vi "IV_Sweep_program1.vi"() -> ()   [LabVIEW 2013]
doc: "I. Description:\nThis example demonstrates how to continuously acquire and generate data at the same time, synchronized with one another.\n\nII. Instructions for Running:\n1. Select the physical channel to correspond to where your signal is input on the DAQ device. Also, select the corresponding channel for where your signal is being generated.\n2. Enter the minimum and maximum voltage ranges.\nNote: For better accuracy try to match the input range to the expected voltage level of the measured signal.\n3. Set the sample rate of the acquisition.\nNote: The rate should be at least twice as fast as the maximum frequency component of the signal being acquired. \n6. Select the Rate for the generation\n7. Select what type of signal to generate and the amplitude.\nNote: This example requires two DMA channels to run. If your hardware does not support two DMA channels, you need to set the Data Transfer Mechanism property for the Analog Output Task to use \"Interrupts\". The Data Transfer Mechanism property is located in the DAQmx Channel Property hierarchy at:\n\nDAQmx Channel Property Node>>Analog Output>>General Properties>>Advanced>>Data Transfer and Memory>>Data Transfer Mechanism\n\nRefer to your device documentation to determine how many DMA channels are supported for your hardware.\n\nIII. Block Diagram Steps:\n1. Create an analog input voltage channel. Also, create an analog output voltage channel.\n2. Set the rate for the sample clock. Additionally, define the sample mode to be continuous. Also, set the sample clock rate for the signal generation.\n2a. Call the Get Terminal Name with Device Prefix VI. This will take a Task and a terminal and create a properly formatted device + terminal name to use as the source of the Trigger.\n3. Define the parameters for a Digital Edge Start Trigger. Set the Analog output to trigger off the AI Start Trigger. This is an internal trigger signal.\n4. Use the Basic Function Generator VI to create the signal to be generated.\n5. Call the Start VI to arm the two functions. Make sure the analog output is armed before the analog input. This will ensure both will start at the same time.\n6. Read the waveform data in a loop until the user hits the stop button or an error occurs. The Is Task Done? VI is used to check for errors in the Analog Output Task.\n7. Call the Clear VI to Clear the Task\n8. Use the popup dialog box to display an error if any.\n\nIV. I/O Connections Overview:\nMake sure your signal input/output terminals match the Physical Channel I/O controls."
uses:
  <vilib>/Utility/error.llb/DialogType.ctl
  <vilib>/DAQmx/read.llb/DAQmx Read (Analog 1D DBL NChan 1Samp).vi
  <vilib>/DAQmx/write.llb/DAQmx Write (Analog DBL 1Chan 1Samp).vi
  <vilib>/DAQmx/create/channels.llb/DAQmx Create Channel (AO-Voltage-Basic).vi
  <vilib>/DAQmx/create/channels.llb/DAQmx Create Channel (AI-Voltage-Basic).vi
  <vilib>/DAQmx/configure/timing.llb/DAQmx Timing (Sample Clock).vi
  <vilib>/DAQmx/miscellaneous.llb/DAQmx Fill In Error Info.vi
  <vilib>/Utility/file.llb/Write To Spreadsheet File (DBL).vi
  <vilib>/Utility/file.llb/Write To Spreadsheet File (I64).vi
panel:
  out "Numeric":i32
  out "x/y":dbl
  in  "Sweep Amplitude":dbl=1.0
  in  "Stop Sweep":bool
  out "Connections 2":string="AI0=Current\nAI1=Bias\nAI2=dI/dV\nAI3=d2I/dV2\nAI4=X-Axis\nAI5=Z-Axis\n"
  out "Connections":string="AO0=Bias\nAO1=Z-axis\nAO2=X-Axis\nAO3=NA"
  in  "Columns":string
  out "Save Indicator":bool
  in  "Update Bias":bool
  in  "Save IV":bool
  in  "Save Decay":bool
  in  "Sweep Bias":bool
  in  "Step Z":bool
  in  "Comment":string="Molecule=C8\nGain=10nA\nBias Gain=div/1\nSweep Freq.=0.005Hz\nRef. Bias=5mV\nRef. Freq=4.33kHz\nGain LIA1=0.5mV\nTC LIA1=300ms\nGain LIA2=\nTC LIA2=\nLIA1=EGG"
  in  "Number Recorded":i32
  in  "DATA Filename":string="Data_"
  in  "Data Directory":path=path "E:/Research/Data"
  out "d2I/dV2":cluster{dbl[], dbl[]}(graph)
  out "dI/dV":cluster{dbl[], dbl[]}(graph)
  out "IV":cluster{dbl[], dbl[]}(graph)
  in  "# Samples":i32=2000
  in  "Frequency (Hz)":dbl=1.0
  in  "stop 3":bool
  in  "Bias":dbl caption="Bias Start Point" step=0.1 format="%_3g"
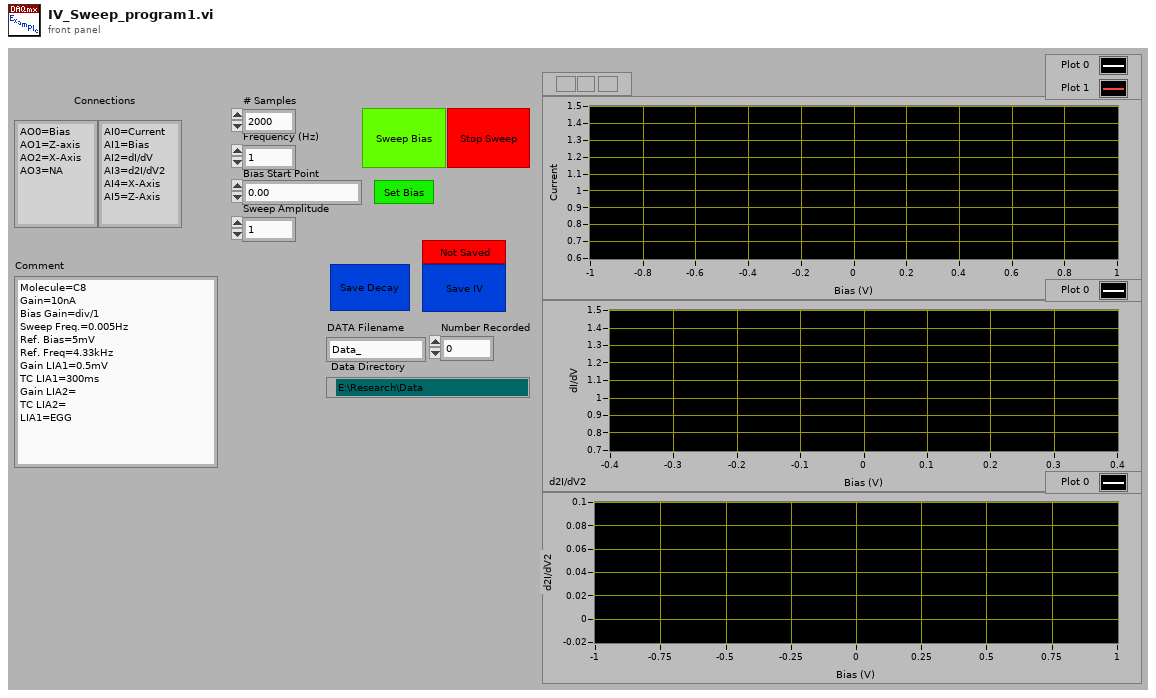
[diagram p1: front panel]
types:
  T1 = enum16{"open", "replace", "create", "open or create", "replace or create", "replace or create with confirmation"}
  T2 = typedef "DialogType.ctl" = u16
  T3 = cluster{dbl[], dbl[], dbl[], dbl[], dbl[], dbl[], dbl[]}
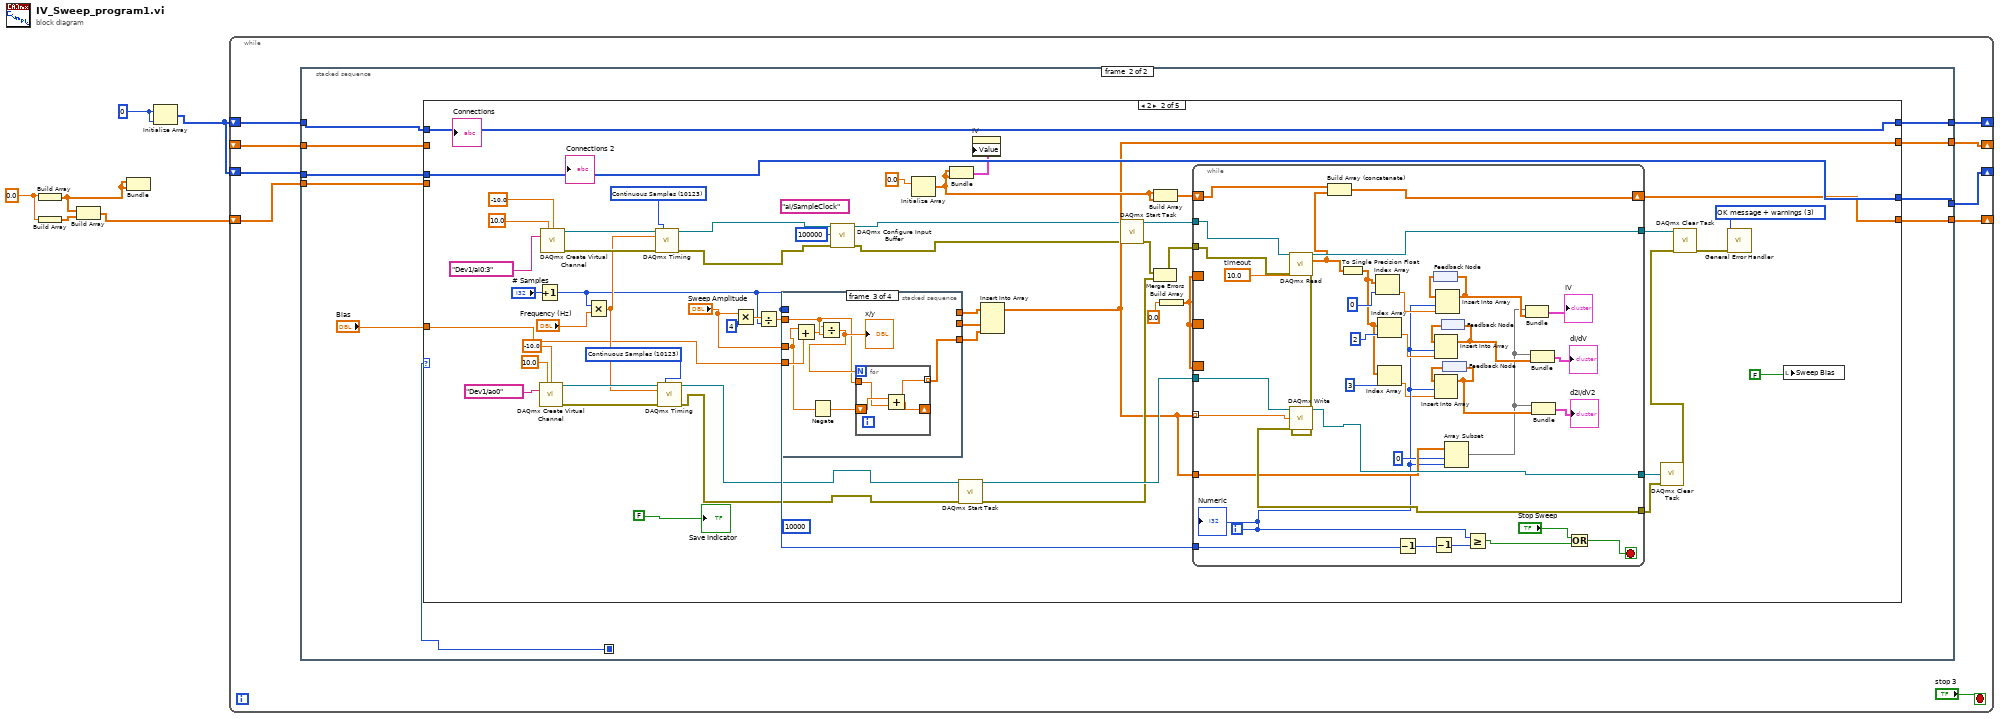
[diagram p0: block diagram]
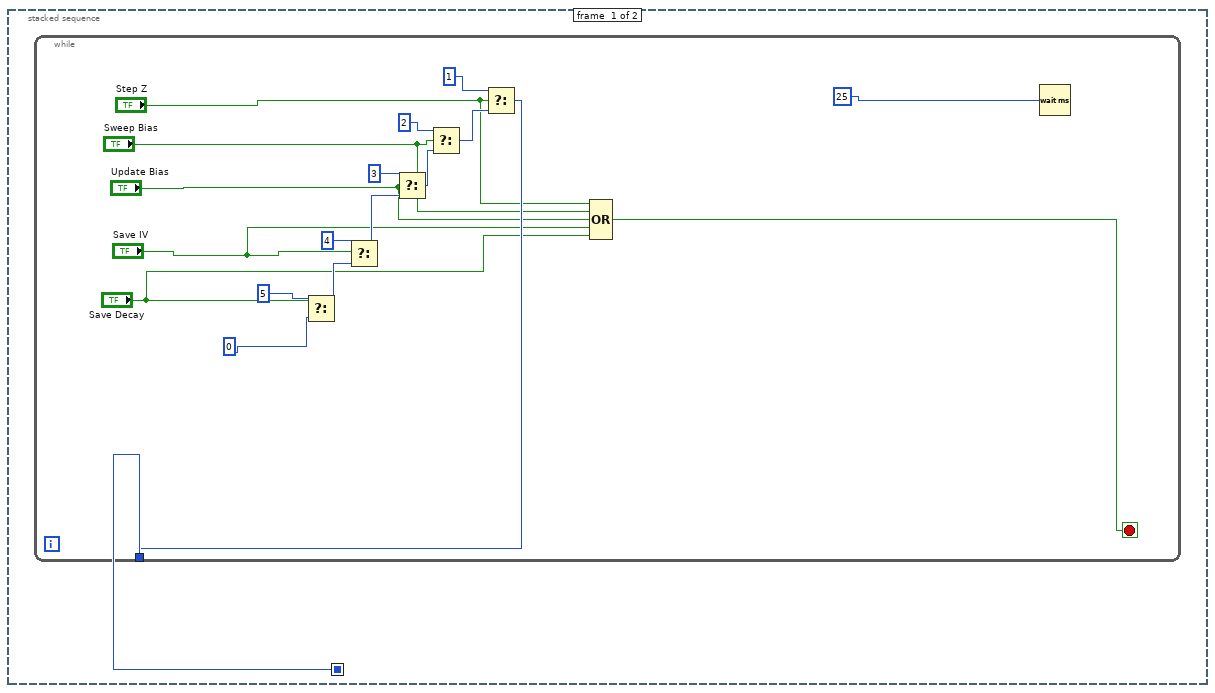
[diagram p2: hidden frame]
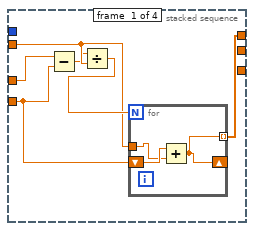
[diagram p4: hidden frame]
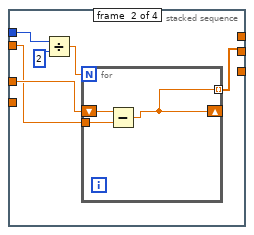
[diagram p5: hidden frame]
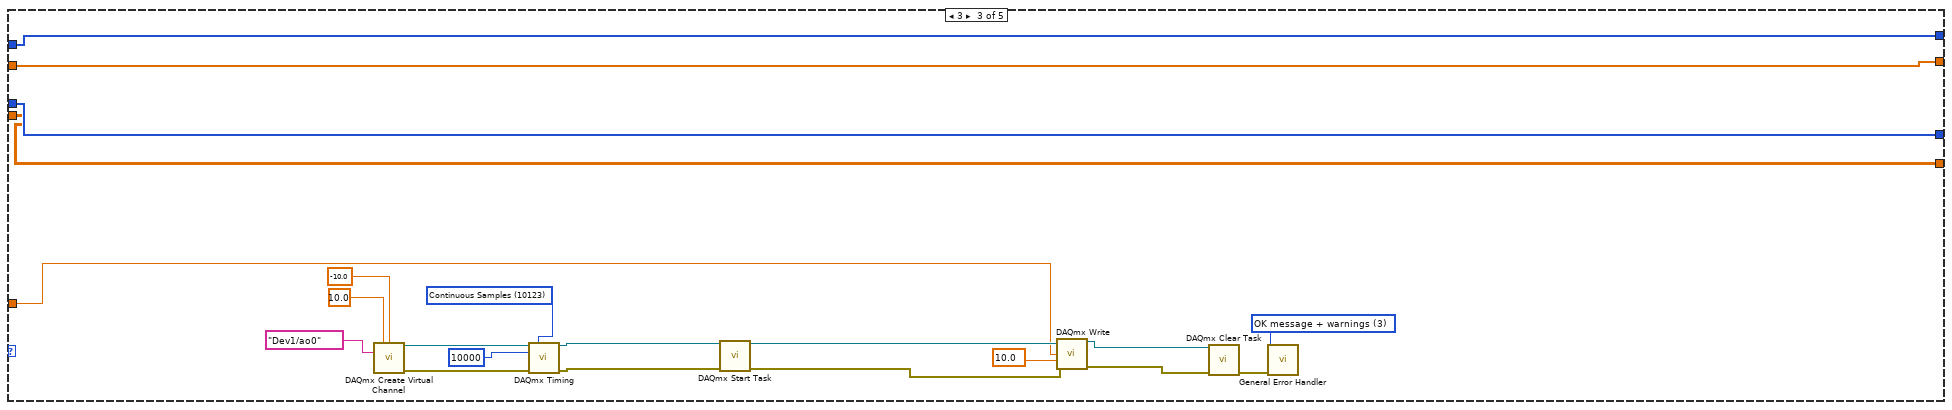
[diagram p7: hidden frame]
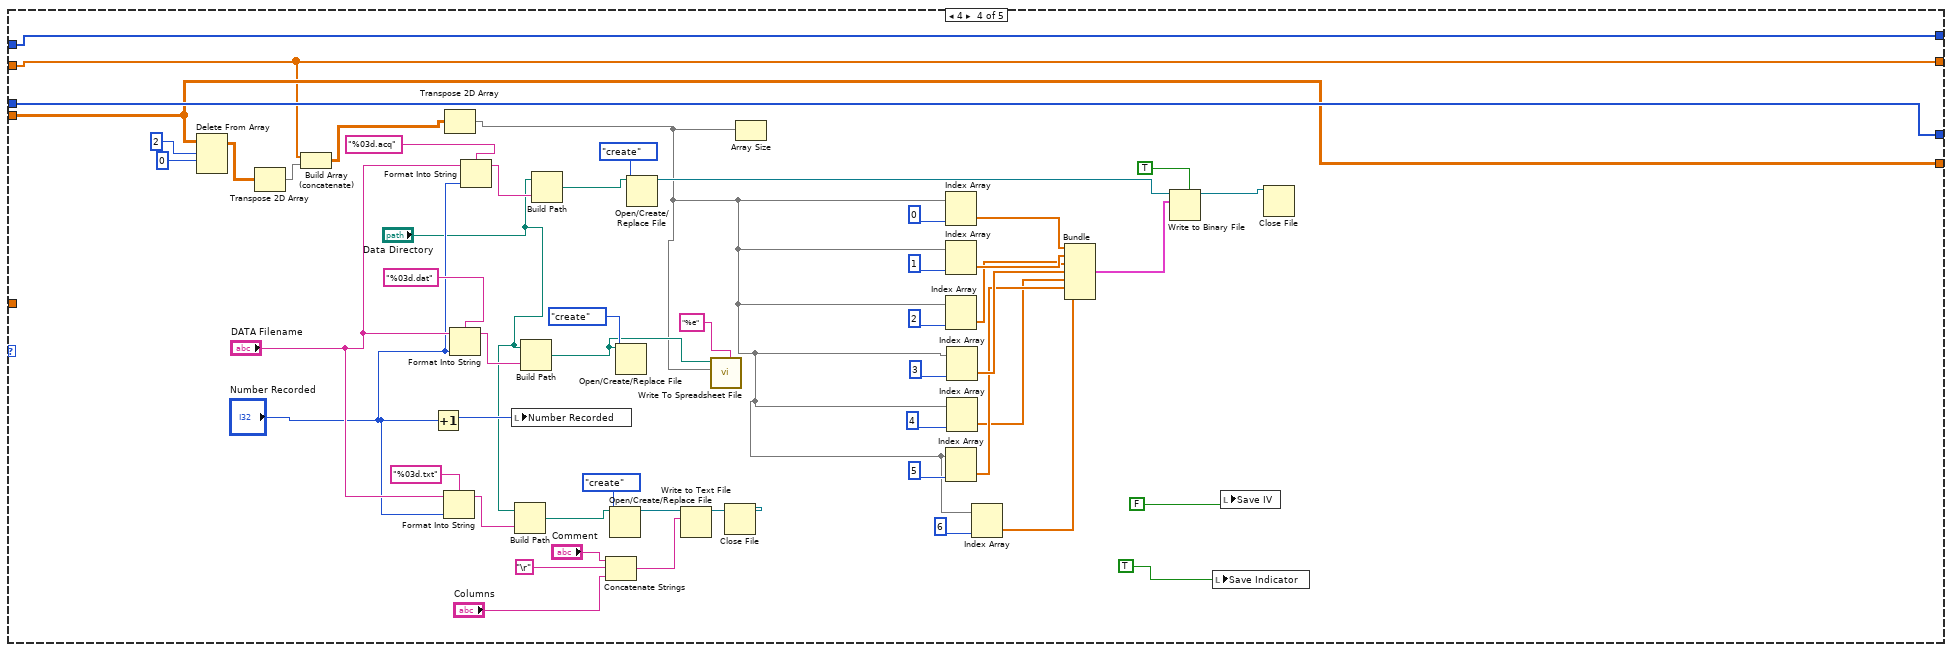
[diagram p8: hidden frame]
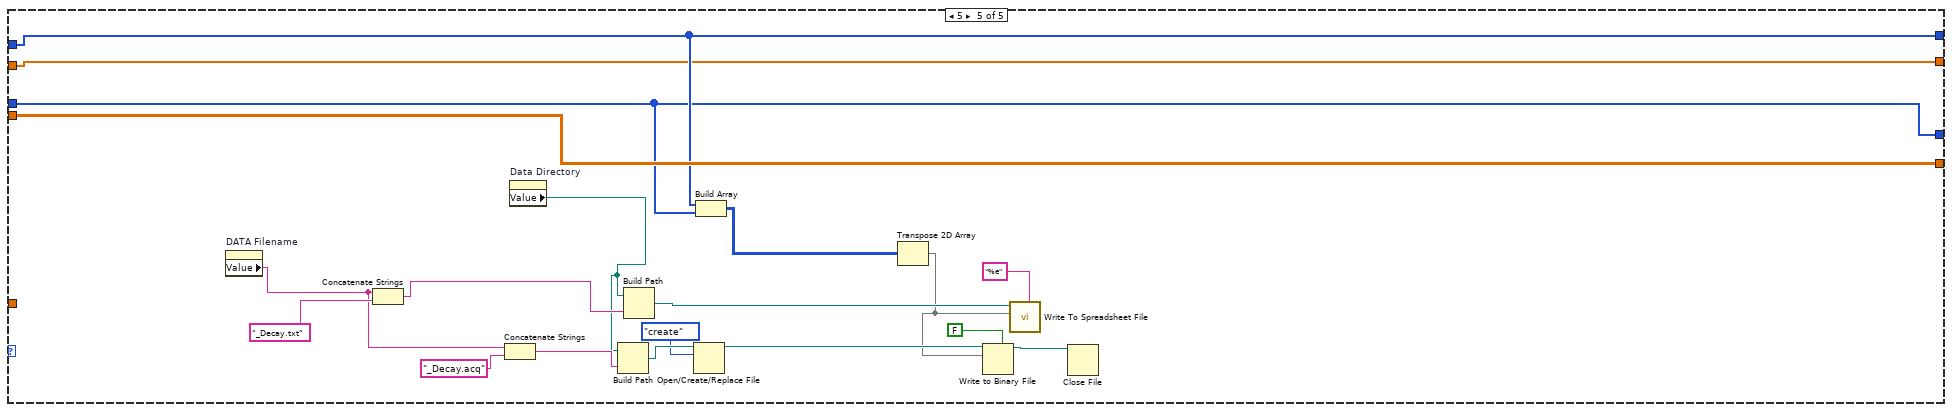
[diagram p9: hidden frame]
diagram:
  w2 = 0
  w6 = 0.0
  n1 = Build Array(w6) -> (w3:dbl[])
  n2 = Build Array(w6) -> (w5:dbl[])
  n3 = Build Array(w3, w5) -> (w4:dbl[][])
  n4 = Bundle(w3, w3) -> ()  [unwired: 1 in, 1 out]
  n5 = Initialize Array(w2, w2) -> (w1:i32[])
  n6 = while {
    shift-right: [w13] -> _
    shift-left: w1 -> [w14]
    shift-right: [w11] -> _
    shift-left: w1 -> [w12]
    shift-right: [w9] -> _
    shift-left: w4 -> [w10]
    shift-right: [w7] -> _
    shift-left: _ -> [w8]
    stop <- "stop 3" stop-if-true
    n7 = stacked-sequence {
      seq-local: [w16 _] -> [_ w44]
      tunnel: w14 -> [_ w43]
      tunnel: [_ w42] -> w13
      tunnel: w12 -> [_ w40]
      tunnel: [_ w39] -> w11
      tunnel: w10 -> [_ w38]
      tunnel: [_ w37] -> w9
      tunnel: w8 -> [_ w36]
      tunnel: [_ w35] -> w7
      frame #0 {
        n8 = while {
          tunnel: [w25] -> w16
          stop <- w24 stop-if-true
          n9 = Select(t=5, s="Save Decay", f=0) -> (s? t:f=w30:i32)
          n10 = Select(t=4, s="Save IV", f=w30) -> (s? t:f=w29:i32)
          n11 = Select(t=3, s="Update Bias", f=w29) -> (s? t:f=w27:i32)
          n12 = Select(t=2, s="Sweep Bias", f=w27) -> (s? t:f=w34:i32)
          n13 = Select(t=1, s="Step Z", f=w34) -> (s? t:f=w25:i32)
          n14 = Compound Arithmetic op=OR("Step Z", "Sweep Bias", "Update Bias", "Save IV", "Save Decay") -> (w24:bool)
          n15 = Wait (ms)(milliseconds to wait=25) -> ()  [unwired: 1 out]
        }
      }
      frame #1 {
        n16 = case shown="2" w44 {
          tunnel: w43 -> [w48 w86 w172 w237 w258]
          tunnel: [w48 w86 w172 w237 w258] -> w42
          tunnel: "Bias" -> [_ w72 w178 _ _]
          tunnel: w40 -> [w47 w83 w173 w238 w259]
          tunnel: [w47 w83 w173 w238 w259] -> w39
          tunnel: w38 -> [w46 _ w170 w217 w260]
          tunnel: [w46 w64 w170 w217 w260] -> w37
          tunnel: [w45 w56 w169 w215 w243] -> w35
          tunnel: w36 -> [w45 _ w169 w215 w243]
          frame 0, Default {
          }
          frame 2 {
            (unwired) 10000
            w81 = 10123 items=["Finite Samples"=10178, "Continuous Samples"=10123, "Hardware Timed Single Point"=12522] ("sample mode")
            w82 = 10123 items=["Finite Samples"=10178, "Continuous Samples"=10123, "Hardware Timed Single Point"=12522] ("sample mode")
            (unwired) "ai/SampleClock" ("terminal")
            w91 = T2 3 items=["no dialog", "OK message", "continue or stop message", "OK message + warnings", "continue/stop + warnings"] ("type of dialog (OK msg:1)")
            n17 = Increment(x="# Samples") -> (x+1=w62:i32)
            n18 = call-poly <vilib>:"DAQmx Create Virtual Channel.vi"("maximum value"=10.0, "minimum value"=-10.0, "physical channels"=tag "Dev1/ao0") -> ("task out"=w94:refnum<k21>, "error out"=w93:errorcluster)  [unwired: 11 in]
            n19 = call-poly <vilib>:"DAQmx Create Virtual Channel.vi"("maximum value"=10.0 ("Maximum Value"), "minimum value"=-10.0 ("Minimum Value"), "physical channels"=tag "Dev1/ai0:3" ("Physical Channel")) -> ("task out"=w98:refnum<k21>, "error out"=w99:errorcluster)  [unwired: 11 in]
            n20 = Multiply(x=w62, y="Frequency (Hz)") -> (x*y=w85:dbl)
            n21 = call-poly <vilib>:"DAQmx Timing.vi"("task/channels in"=w98, "sample mode"=w81, "rate"=w85, "error in"=w99) -> ("task out"=w50:refnum<k21>, "error out"=w52:errorcluster)  [unwired: 10 in]
            n22 = call-poly <vilib>:"DAQmx Timing.vi"("task/channels in"=w94, "sample mode"=w82, "rate"=w85, "error in"=w93) -> ("task out"=w54:refnum<k21>, "error out"=w53:errorcluster)  [unwired: 10 in]
            n23 = Multiply(x="Sweep Amplitude", y=4) -> (x*y=w70:dbl)
            n24 = Divide(x=w70, y=w62) -> (x/y=w69:dbl)
            n25 = stacked-sequence {
              tunnel: "Sweep Amplitude" -> [w146 w152 w160 _]
              tunnel: w72 -> [w144 _ w164 _]
              tunnel: w69 -> [w142 w151 w162 _]
              tunnel: [w143 _ _ _] -> w68
              tunnel: w62 -> [_ w155 _ _]
              tunnel: [_ w150 _ _] -> w67
              tunnel: [_ _ w163 _] -> w66
              frame #0 {
                n26 = Subtract(x=w146, y=w144) -> (x-y=w141:dbl)
                n27 = Divide(x=w141, y=w142) -> (x/y=w145:dbl)
                n28 = for {
                  N: w145 -> [_]
                  tunnel: w142 -> [w148]
                  shift-right: [w147] -> _
                  shift-left: w144 -> [w149]
                  tunnel: [w147] -> w143 mode=indexing
                  n29 = Add(x=w149, y=w148) -> (x+y=w147:dbl)
                }
              }
              frame #1 {
                n30 = Divide(x=w155, y=2) -> (x/y=w153:dbl)
                n31 = for {
                  N: w153 -> [_]
                  tunnel: w151 -> [w157]
                  shift-right: [w156] -> _
                  shift-left: w152 -> [w158]
                  tunnel: [w156] -> w150 mode=indexing
                  n32 = Subtract(x=w158, y=w157) -> (x-y=w156:dbl)
                }
              }
              frame #2 {
                n33 = Add(x=w160, y=w164) -> (x+y=w161:dbl)
                n34 = Negate(x=w160) -> (-x=w159:dbl)
                n35 = Divide(x=w161, y=w162) -> (x/y=w165:dbl)
                "x/y" <- w165
                n36 = for {
                  N: w165 -> [_]
                  tunnel: w162 -> [w167]
                  shift-right: [w166] -> _
                  shift-left: w159 -> [w168]
                  tunnel: [w166] -> w163 mode=indexing
                  n37 = Add(x=w168, y=w167) -> (x+y=w166:dbl)
                }
              }
              frame #3 {
              }
            }
            n38 = call <vilib>:"DAQmx Configure Input Buffer.vi"("task/channels in"=w50, "buffer size (in samples per channel)"=100000, "error in"=w52) -> ("task out"=w49:refnum<k21>, "error out"=w51:errorcluster)  [unwired: 11 in]
            n39 = Initialize Array(0.0) -> (w61:dbl[])  [unwired: 1 in]
            n40 = Bundle(w61, w61) -> (w60:cluster{dbl[], dbl[]})  [unwired: 1 in]
            n41 = call <vilib>:"DAQmx Start Task.vi"("task/channels in"=w54, "error in"=w53) -> ("task out"=w80:refnum<k21>, "error out"=w76:errorcluster)  [unwired: 12 in]
            n42 = property on="IV" class="XYGraph (strict)"("Value"=w60) -> ()  [unwired: 2 in, 2 out]
            n43 = Insert Into Array(array=w68, new element #1=w67, new element #2=w66) -> (w56:dbl[])  [unwired: 1 in]
            n44 = call <vilib>:"DAQmx Start Task.vi"("task/channels in"=w49, "error in"=w51) -> ("task out"=w78:refnum<k21>, "error out"=w77:errorcluster)  [unwired: 12 in]
            n45 = Merge Errors(w77, w76) -> (w79:errorcluster)
            n46 = Build Array(w61, w61) -> (w63:dbl[][])
            n47 = Build Array(0.0) -> (w58:dbl[])
            n48 = while {
              tunnel: [w132] -> w100
              tunnel: [w135] -> w92
              tunnel: [w134] -> w89
              tunnel: w62 -> [w106]
              tunnel: w56 -> [w111] mode=indexing
              tunnel: w80 -> [w137]
              tunnel: w78 -> [w140]
              tunnel: w79 -> [w139]
              shift-right: [w112] -> w64
              shift-left: w63 -> [w133]
              tunnel: w56 -> [w130]
              border: w58 -> [_]
              border: w58 -> [_]
              border: w58 -> [_]
              i -> [w107]
              stop <- w108 stop-if-true
              w136 = 10.0  # timeout
              n49 = call-poly <vilib>:"DAQmx Read.vi"("task/channels in"=w140, "timeout"=w136, "error in"=w139) -> ("task out"=w132:refnum<k21>, "data"=w114:dbl[], "error out"=w138:errorcluster)  [unwired: 10 in]
              n50 = call-poly <vilib>:"DAQmx Write.vi"("task/channels in"=w137, "data"=w111, "error in"=w138) -> ("task out"=w135:refnum<k21>, "error out"=w134:errorcluster)  [unwired: 10 in, 1 out]
              n51 = Build Array (concatenate)(w133, w114) -> (w112:dbl[][])
              n52 = To Single Precision Float(number=w114) -> (single precision float=w113:sgl[])
              n53 = Index Array(array=w113, index=0) -> (element=w127:sgl)
              n54 = Index Array(array=w113, index=2) -> (element=w123:sgl)
              n55 = Index Array(array=w113, index=3) -> (element=w103:sgl)
              n56 = Decrement(x=w106) -> (x-1=w104:i32)
              n57 = Decrement(x=w104) -> (x-1=w105:i32)
              n58 = feedback #1() -> (w126:dbl[])
              n59 = Insert Into Array(array=w126, index=w107, new element=w127) -> (w128:dbl[])
              n60 = feedback-in #1(w128) -> ()
              n61 = feedback #2() -> (w122:dbl[])
              n62 = Insert Into Array(array=w122, index=w107, new element=w123) -> (w120:dbl[])
              n63 = feedback-in #2(w120) -> ()
              n64 = feedback #3() -> (w121:dbl[])
              n65 = Insert Into Array(array=w121, index=w107, new element=w103) -> (w119:dbl[])
              n66 = feedback-in #3(w119) -> ()
              n67 = Array Subset(array=w130, index=0, length=w107) -> (w118:dbl[])
              n68 = Greater Or Equal?(x=w107, y=w105) -> (x >= y?=w109:bool)
              n69 = Bundle(w118, w128) -> (→"IV":cluster{dbl[], dbl[]})  [unwired: 1 in]
              n70 = Bundle(w118, w120) -> (→"dI/dV":cluster{dbl[], dbl[]})  [unwired: 1 in]
              n71 = Bundle(w118, w119) -> (→"d2I/dV2":cluster{dbl[], dbl[]})  [unwired: 1 in]
              n72 = Or(x="Stop Sweep", y=w109) -> (x .or. y?=w108:bool)
              "Numeric" <- w107
            }
            n73 = call <vilib>:"DAQmx Clear Task.vi"("task in"=w92, "error in"=w89) -> ("error out"=w88:errorcluster)  [unwired: 13 in]
            n74 = call <vilib>:"DAQmx Clear Task.vi"("task in"=w100, "error in"=w88) -> ("error out"=w87:errorcluster)  [unwired: 13 in]
            n75 = call <vilib>:"General Error Handler.vi"("type of dialog (OK msg:1)"=w91, "error in (no error)"=w87) -> ()  [unwired: 9 in, 5 out]
            n76 = local write "Sweep Bias"(FALSE) -> ()
            "Save Indicator" <- FALSE
          }
          frame 3 {
            w177 = T2 3 items=["no dialog", "OK message", "continue or stop message", "OK message + warnings", "continue/stop + warnings"] ("type of dialog (OK msg:1)")
            w183 = 10123 items=["Finite Samples"=10178, "Continuous Samples"=10123, "Hardware Timed Single Point"=12522] ("sample mode")
            n77 = call-poly <vilib>:"DAQmx Create Virtual Channel.vi"("maximum value"=10.0 ("maximum value 2"), "minimum value"=-10.0 ("minimum value 2"), "physical channels"=tag "Dev1/ao0" ("physical channels 2")) -> ("task out"=w186:refnum<k21>, "error out"=w185:errorcluster)  [unwired: 11 in]
            n78 = call-poly <vilib>:"DAQmx Timing.vi"("task/channels in"=w186, "sample mode"=w183, "rate"=10000, "error in"=w185) -> ("task out"=w182:refnum<k21>, "error out"=w181:errorcluster)  [unwired: 10 in]
            n79 = call <vilib>:"DAQmx Start Task.vi"("task/channels in"=w182, "error in"=w181) -> ("task out"=w180:refnum<k21>, "error out"=w179:errorcluster)  [unwired: 12 in]
            n80 = call-poly <vilib>:"DAQmx Write.vi"("task/channels in"=w180, "data"=w178, "timeout"=10.0 ("Wirite Timeout"), "error in"=w179) -> ("task out"=w175:refnum<k21>, "error out"=w174:errorcluster)  [unwired: 9 in, 1 out]
            n81 = call <vilib>:"DAQmx Clear Task.vi"("task in"=w175, "error in"=w174) -> ("error out"=w176:errorcluster)  [unwired: 13 in]
            n82 = call <vilib>:"General Error Handler.vi"("type of dialog (OK msg:1)"=w177, "error in (no error)"=w176) -> ()  [unwired: 9 in, 5 out]
          }
          frame 4 {
            n83 = Delete From Array(array=w217, length=2, index (row)=0) -> (array with subset deleted=w214:dbl[][])  [unwired: 1 in, 1 out]
            n84 = Transpose 2D Array(2D array=w214) -> (transposed array=w213:dbl[][])
            n85 = Build Array (concatenate)(w215, w213) -> (w212:dbl[][])
            n86 = Increment(x="Number Recorded") -> (x+1=w240:i32)
            n87 = Format Into String(format string="%03d.txt", initial string="DATA Filename", "Number Recorded") -> (resulting string=w228:string)  [unwired: 1 in, 1 out]
            n88 = Transpose 2D Array(2D array=w212) -> (transposed array=w199:dbl[][])
            n89 = Format Into String(format string="%03d.dat", initial string="DATA Filename", "Number Recorded") -> (resulting string=w242:string)  [unwired: 1 in, 1 out]
            n90 = Format Into String(format string="%03d.acq", initial string="DATA Filename", "Number Recorded") -> (resulting string=w235:string)  [unwired: 1 in, 1 out]
            n91 = local write "Number Recorded"(w240) -> ()
            n92 = Build Path(base path="Data Directory", name or relative path=w228) -> (appended path=w226:path)
            n93 = Build Path(base path="Data Directory", name or relative path=w242) -> (appended path=w239:path)
            n94 = Build Path(base path="Data Directory", name or relative path=w235) -> (appended path=w233:path)
            n95 = Concatenate Strings("Comment", "\r", "Columns") -> (w209:string)
            n96 = Open/Create/Replace File(file path (use dialog)=w226, operation (0:open)=T1."create") -> (refnum out=w221:refnum<file>)  [unwired: 4 in, 2 out]
            n97 = Open/Create/Replace File(file path (use dialog)=w239, operation (0:open)=T1."create") -> ()  [unwired: 4 in, 3 out]
            n98 = Open/Create/Replace File(file path (use dialog)=w233, operation (0:open)=T1."create") -> (refnum out=w232:refnum<file>)  [unwired: 4 in, 2 out]
            n99 = Write to Text File(file (use dialog)=w221, text=w209) -> (refnum out=w220:refnum<file>)  [unwired: 2 in, 2 out]
            n100 = call-poly <vilib>:"Write To Spreadsheet File.vi"("format (%.3f)"="%e", "2D data"=w199, "file path (dialog if empty)"=w239) -> ()  [unwired: 5 in, 1 out]
            n101 = Close File(refnum=w220) -> ()  [unwired: 1 in, 2 out]
            n102 = Array Size(array=w199) -> ()  [unwired: 1 out]
            n103 = Index Array(array=w199, index (col)=0) -> (element=w198:dbl[])  [unwired: 1 in]
            n104 = Index Array(array=w199, index (col)=1) -> (element=w197:dbl[])  [unwired: 1 in]
            n105 = Index Array(array=w199, index (col)=2) -> (element=w196:dbl[])  [unwired: 1 in]
            n106 = Index Array(array=w199, index (col)=5) -> (element=w194:dbl[])  [unwired: 1 in]
            n107 = Index Array(array=w199, index (col)=3) -> (element=w195:dbl[])  [unwired: 1 in]
            n108 = Index Array(array=w199, index (col)=4) -> (element=w190:dbl[])  [unwired: 1 in]
            n109 = Index Array(array=w199, index (col)=6) -> (element=w193:dbl[])  [unwired: 1 in]
            n110 = Bundle(w198, w197, w196, w195, w190, w194, w193) -> (w192:T3)  [unwired: 1 in]
            n111 = Write to Binary File(file (use dialog)=w232, data=w192, 5:TRUE ("prepend array or string size? (T)")) -> (refnum out=w230:refnum<file>)  [unwired: 3 in, 2 out]
            n112 = local write "Save Indicator"(TRUE) -> ()
            n113 = local write "Save IV"(FALSE) -> ()
            n114 = Close File(refnum=w230) -> ()  [unwired: 1 in, 2 out]
          }
          frame 5 {
            n115 = property on="DATA Filename" class="Str"() -> ("Value"=w253:string)  [unwired: 2 in, 2 out]
            n116 = Concatenate Strings(w253, "_Decay.txt") -> (w257:string)
            n117 = Concatenate Strings(w253, "_Decay.acq") -> (w251:string)
            n118 = property on="Data Directory" class="Path"() -> ("Value"=w250:path)  [unwired: 2 in, 2 out]
            n119 = Build Path(base path=w250, name or relative path=w251) -> (appended path=w249:path)
            n120 = Build Path(base path=w250, name or relative path=w257) -> (appended path=w256:path)
            n121 = Open/Create/Replace File(file path (use dialog)=w249, operation (0:open)=T1."create") -> (refnum out=w255:refnum<file>)  [unwired: 4 in, 2 out]
            n122 = Build Array(w259, w258) -> (w246:i32[][])
            n123 = Transpose 2D Array(2D array=w246) -> (transposed array=w245:i32[][])
            n124 = Write to Binary File(file (use dialog)=w255, data=w245, 5:FALSE ("prepend array or string size? (T)")) -> (refnum out=w254:refnum<file>)  [unwired: 3 in, 2 out]
            n125 = call-poly <vilib>:"Write To Spreadsheet File.vi"("format (%d)"="%e", "2D data"=w245, "file path (dialog if empty)"=w256) -> ()  [unwired: 5 in, 1 out]
            n126 = Close File(refnum=w254) -> ()  [unwired: 1 in, 2 out]
          }
        }
      }
    }
  }
